vi "EnaTrigTmstmp.vi"(8 "error in (no error)":errorcluster, 10 "clEnaTrigTmstmp":T1, 11 "PXI_MultiTrig in":refnum<class "PXI_MultiTrig.lvclass">) -> (0 "error out":errorcluster, 3 "PXI_MultiTrig out":refnum<class "PXI_MultiTrig.lvclass">)   [LabVIEW 2018, in "SyncPlugins.lvlib" / "PXI_MultiTrig.lvclass"]
uses:
  PXI_MultiTrig.lvclass
  SyncPluginBase/Typedefs/clEnaTrigTmstmp.ctl
  PXI_MultiTrig.lvclass/PXI_MultiTrig.ctl
  Accessors/Write RefClkSession.vi
  Accessors/Write Triggers.vi
  Accessors/Read RefClkSession.vi
  Accessors/Read Triggers.vi
  <vilib>/Utility/error.llb/Error Cluster From Error Code.vi
  <vilib>/ErrorRing/Error Ring.xnode
  SyncPluginBase/SyncPluginBase.lvclass
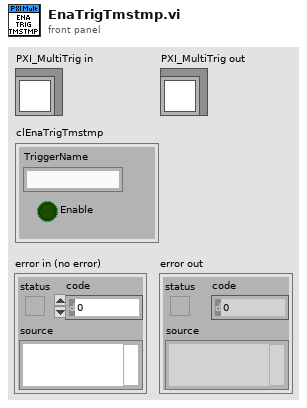
[diagram p1: front panel]
types:
  T1 = typedef "SyncPlugins.lvlib/SyncPluginBase.lvclass/clEnaTrigTmstmp.ctl" = cluster{"TriggerName":string, "Enable":bool}
  T2 = typedef "SyncPlugins.lvlib/PXI_MultiTrig.lvclass/clTrigger.ctl" = cluster{"Name":string, "DestTerm":string, "SrcTerm":string, "SyncClk":string, "Edge":i32, "Invert?":i32, "Initiated":bool, "Type":string, "TrigTime":bool}
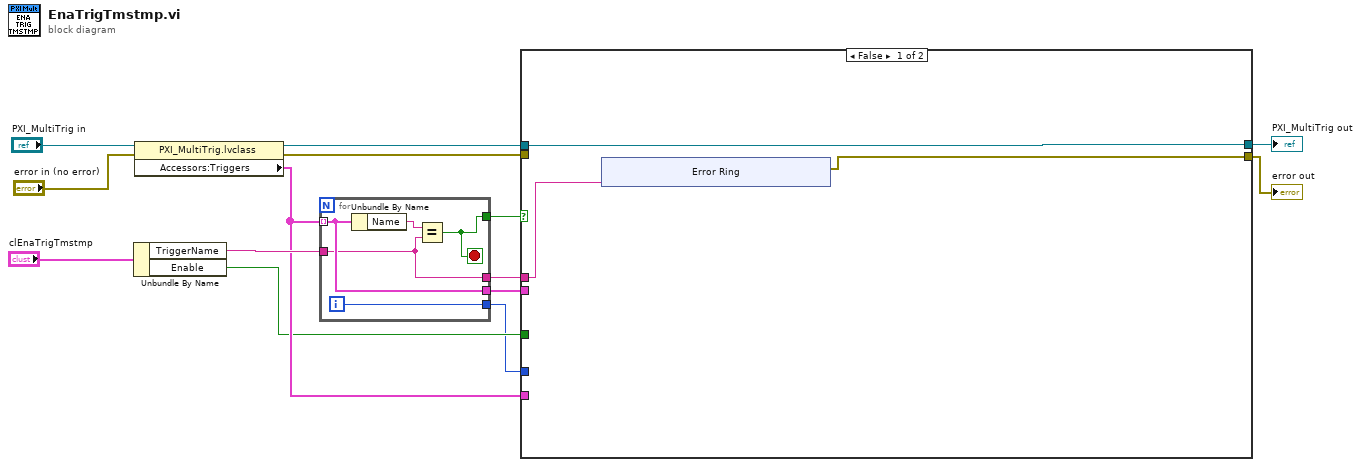
[diagram p0: block diagram]
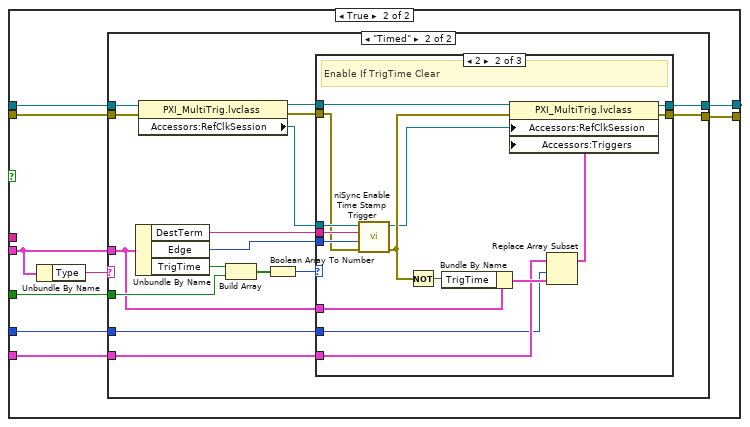
[diagram p2: hidden frame]
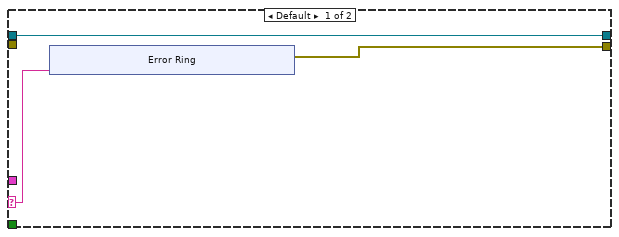
[diagram p3: hidden frame]
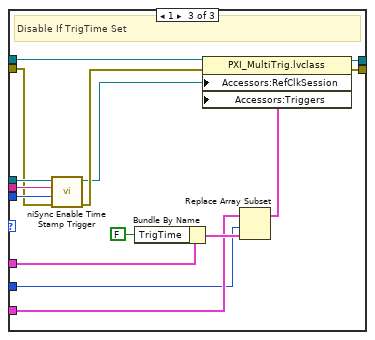
[diagram p5: hidden frame]
diagram:
  n1 = Unbundle By Name("clEnaTrigTmstmp") -> ("TriggerName"=w12:string, "Enable"=w5:bool)
  n2 = property class="PXI_MultiTrig.lvclass"(reference="PXI_MultiTrig in", error in="error in (no error)") -> (reference out=w10:refnum<class "PXI_MultiTrig.lvclass">, error out=w9:errorcluster, "Accessors:Triggers"=w6:T2[])
  n3 = for {
    tunnel: w6 -> [w18] mode=indexing
    tunnel: [w18] -> w7
    tunnel: [w15] -> w11
    tunnel: [w17] -> w4
    tunnel: w12 -> [w16]
    tunnel: [w16] -> w8
    i -> [w17]
    stop <- w15 stop-if-true
    n4 = Unbundle By Name(w18) -> ("Name"=w19:string)
    n5 = Equal?(x=w19, y=w16) -> (x = y?=w15:bool)
  }
  n6 = case shown="False" w11 {
    tunnel: w10 -> [w22 w36]
    tunnel: w9 -> [_ w34]
    tunnel: [w22 w35] -> w2
    tunnel: w8 -> [w21 _]
    tunnel: [w20 w37] -> w3
    tunnel: w7 -> [_ w33]
    tunnel: w6 -> [_ w32]
    tunnel: w5 -> [_ w31]
    tunnel: w4 -> [_ w30]
    frame False {
      n7 = xnode "Error Ring"("parameter 0"=w21) -> ("error out"=w20:errorcluster)
    }
    frame True {
      n8 = Unbundle By Name(w33) -> ("Type"=w38:string)
      n9 = case shown="\"Timed\"" w38 {
        selector: w38 -> [w40 _]
        tunnel: [w39 w49] -> w37
        tunnel: w36 -> [w41 w64]
        tunnel: [w41 w50] -> w35
        tunnel: w34 -> [_ w63]
        tunnel: w33 -> [_ w52]
        tunnel: w32 -> [_ w53]
        tunnel: w31 -> [_ w61]
        tunnel: w30 -> [_ w51]
        frame Default {
          n10 = xnode "Error Ring"("parameter 0"=w40) -> ("error out"=w39:errorcluster)
        }
        frame "Timed" {
          n11 = Unbundle By Name(w52) -> ("DestTerm"=w57:string, "Edge"=w56:i32, "TrigTime"=w62:bool)
          n12 = property class="PXI_MultiTrig.lvclass"(reference=w64, error in=w63) -> (reference out=w55:refnum<class "PXI_MultiTrig.lvclass">, error out=w54:errorcluster, "Accessors:RefClkSession"=w58:refnum<k15>)
          n13 = Build Array(w62, w61) -> (w60:bool[])
          n14 = Boolean Array To Number(Boolean array=w60) -> (number=w59:u32)
          n15 = case shown="2" w59 {
            tunnel: w58 -> [_ w81 w96]
            tunnel: w57 -> [_ w80 w95]
            tunnel: w56 -> [_ w79 w94]
            tunnel: w55 -> [w66 w75 w91]
            tunnel: w54 -> [w65 w78 w93]
            tunnel: w53 -> [_ w71 w87]
            tunnel: w52 -> [_ w77 w92]
            tunnel: w51 -> [_ w70 w86]
            tunnel: [w66 w68 w83] -> w50
            tunnel: [w65 w67 w82] -> w49
            frame 0, Default {
            }
            frame 2 {
              # "Enable If TrigTime Clear"
              n16 = call <instrlib>:"niSync Enable Time Stamp Trigger.vi"("error in (no error)"=w78, "active edge"=w79, "terminal"=w80, "instrument handle"=w81) -> ("error out"=w74:errorcluster, "instrument handle out"=w73:refnum<k15>)  [unwired: 5 in]
              n17 = Not(x=w74) -> (.not. x?=w76:bool)
              n18 = Bundle By Name(cluster=w77, "TrigTime"=w76) -> (w72:T2)
              n19 = Replace Array Subset(array=w71, new element=w72, index=w70) -> (w69:T2[])
              n20 = property class="PXI_MultiTrig.lvclass"(reference=w75, error in=w74, "Accessors:RefClkSession"=w73, "Accessors:Triggers"=w69) -> (reference out=w68:refnum<class "PXI_MultiTrig.lvclass">, error out=w67:errorcluster)
            }
            frame 1 {
              # "Disable If TrigTime Set"
              n21 = call <instrlib>:"niSync Enable Time Stamp Trigger.vi"("error in (no error)"=w93, "active edge"=w94, "terminal"=w95, "instrument handle"=w96) -> ("error out"=w90:errorcluster, "instrument handle out"=w89:refnum<k15>)  [unwired: 5 in]
              n22 = Bundle By Name(cluster=w92, "TrigTime"=FALSE) -> (w88:T2)
              n23 = Replace Array Subset(array=w87, new element=w88, index=w86) -> (w85:T2[])
              n24 = property class="PXI_MultiTrig.lvclass"(reference=w91, error in=w90, "Accessors:RefClkSession"=w89, "Accessors:Triggers"=w85) -> (reference out=w83:refnum<class "PXI_MultiTrig.lvclass">, error out=w82:errorcluster)
            }
          }
        }
      }
    }
  }
  "error out" <- w3
  "PXI_MultiTrig out" <- w2
